vi "GetAcqSeq.vi"(0 "Pre-Looks":i32, 1 "Digitizer Settings":T8={"Digitizer delay (us) "=0.0, "rf points per line"=2048, "lines per plane"=128, "Samp Rate (Hz)"=100000000.0, "Additional dig delay (us)"=0.0, "Voltage Scale"=0.4, "Pre-Looks"=0, "Offset delay (us)"=0.0, "bits A/D"=8, "Avg Num"=1, "DigTimeOut"=5.0, "Rel Dig Delay"=0.0, "Dig Ch"=0, "LeCroyCluster"={"LeCroy Channels"=[TRUE, FALSE, FALSE, FALSE], "LC read pt offset"=0.0, "Sweep Avg"=FALSE}, "Main Digitizer"=enum."NI Digitizer", "Dig Config"=enum."Single channel", "Digitizer ID Cluster"={"Acqiris/Alazar/SP ID"=[], "NI Instr Handles"=[], "LeCroy VISA"="", "GaGe Handle"={"Handle"=0, "Sample size"=0, "Resolution"=0, "Offset"=0, "Channels"=0, "Boards"=0}, "ATS Ref"="ATS9350", "Acqiris Address"=["PCI::INSTR0"], "ADQRef"=refnum, "adq_cu_ptr"=refnum}, "Trigger Settings"={"Trig Source"=1, "Trig Coupling"=0, "Trig Slope"=0, "Level (mV)"=1500.0}, "Bulk Acq"=FALSE, "Bulk Start Indexes"=[], "Data Ref RF"=refnum, "NI ID/Channel"=[], "Total Dig CH"=1, "Xtra Ann Trig delay (us)"=10.0, "Fix Z Delay?"=FALSE, "One Way Transmission?"=FALSE, "Data Ref Log"=refnum} {"Trigger Settings"."Trig Slope" items=["Positive", "Negative"]; "Trigger Settings"."Level (mV)" format="%.2f"; "Trigger Settings"."Trig Coupling" items=["DC 1 MOhm", "AC 1 MOhm", "DC 50 Ohm", "AC 50 Ohm"]; "Trigger Settings"."Trig Source" items=["Chan 1", "External"]; "Rel Dig Delay" format="%.2f"; "DigTimeOut" format="%.2f"; "Avg Num" min=1; "Offset delay (us)" format="%.2f"; "Additional dig delay (us)" format="%.2f"; "Digitizer delay (us)" format="%.2f"}, 3 "Acq Card ID":u32, 6 "Motion Settings":T4={"No Motion?"=FALSE, "Motion System"=enum."NI 735x", "Motion Bd ID"=1, "Motion Profile"="SMAC1", "# Axis"=1, "Reverse Z axis?"=TRUE, "SMAC Axis"=0, "scan pair"=enum."y-(x) scan", "RT fps"=6.0, "Steps per mm"=[1000, 1000, 1000, 1000], "Motor Parameters"={"velocity ct/s"=[10000.0, 10000.0, 10000.0, 50000.0], "accel ct/s^2"=[50000.0, 50000.0, 50000.0, 200000.0]}, "One Way Scan"=FALSE, "Reverse One Way Scan"=FALSE, "Global Position (mm)"=[], "Plane"=0, "Distance between\nscan lines (um)"=0.0, "Distance between\nscan planes (um)"=0.0, "number of scan planes"=1, "Total steps in line"=0, "Xtra plane\ndistance  (um)"=100, "Xtra planes "=1, "Add Axis"=FALSE, "overshoot cts"=200, "BKPT Shift"=0, "Scan Start Time (ms)"=0, "ESP VISA"="GPIB::1::INSTR", "3rd Axis"=1, "GL Ref Out"=refnum, "Galil Address"=""} {"3rd Axis" items=["x", "y", "z", "w"]; "Xtra planes" min=1; "Xtra plane\ndistance  (um)" min=0; "Distance between\nscan planes (um)" format="%.2f"; "Distance between\nscan lines (um)" format="%.2f"; "SMAC Axis" items=["None"=0, "Axis 1"=1, "Axis 2"=2, "Axis 3"=3, "Axis 4"=4, "Axis 5"=5, "Axis 6"=6, "Axis 7"=7, "Axis 8"=8, "Vector Space 1"=17, "Vector Space 2"=18, "Vector Space 3"=19, "Vector Space 4"=20]; "Motion Bd ID" min=1 max=32 step=1}, 7 "errorin":errorcluster, 8 "Numbered File":string, 9 "Divide prf by":i32, 10 "lines per plane":i32, 11 "Channel (1)":i32=1, 12 "Ann Array Params":T1={"Synth Foc?"=FALSE, "Focal Zones"=41, "Switch T/R"=0, "Trans Geometry (mm)"={"Transducer"=0, "Geo Focus"=12.0, "a (radius)"=3.0, "# of rings"=5, "kerf space "=0.1, "Center Freq"=12.0}, "Sub Ap Excite?"=FALSE, "Full Array Scan?"=FALSE, "Xmt/Rcv"={"XMIT"=[TRUE, TRUE, TRUE, TRUE, TRUE], "RCV"=[TRUE, TRUE, TRUE, TRUE, TRUE]}, "PulseSpacing (us)"=0.0, "Xmit Ring"=0, "XMIT CHS"=0, "RCV CHS"=0, "GPU?"=FALSE, "Save TIFF?"=FALSE, "downfactor"=1, "RCV 1CH"=0} {"RCV 1CH" items=["All", "1", "2", "3", "4", "5"]; "Trans Geometry (mm)"."Transducer" items=["6D 12R 40 MHz"=0, "10D 31R 20 MHz"=1, "10D 23R 20 MHz"=2, "6D 23R 40 MHz"=3, "4.5D 10.7R 40 MHz"=4, "9D 23.5R 20 MHz"=5, "9D 25.8R 20MHz"=6, "Enter"=99]; "Switch T/R" min=1 max=5 step=1}, 13 "Rcv Ring":i32, 14 "save?":bool=TRUE, 15 "Reverse?":bool) -> (17 "Raw VGain (scale)":dbl, 18 "Voltage Scale":T12, 20 "Array":i16[][](array[numeric]), 21 "VGain (dB)":dbl, 25 "Synth App Out":i16[][](array[numeric]), 27 "error out":errorcluster)   [LabVIEW 2022 SP3]
uses:
  -DigitizerRoutines/DigitizerSettings.ctl
  -DigitizerRoutines/Digitizer.ctl
  -DigitizerRoutines/DigConfig.ctl
  -DigitizerRoutines/DigitizerID.ctl
  C:/Windows/System32/ADQAPI_dotNet_helper.dll
  Motion Controllers/NI_controller/-NI_MotionRoutines/MotionParameters.ctl
  Motion Controllers/NI_controller/-NI_MotionRoutines/MotionSys.ctl
  Motion Controllers/-MotionRoutines/ScanAxis.ctl
  Motion Controllers/-MotionRoutines/3rdAxis.ctl
  Annular Array/-AnnularRoutines/AnnularArray.ctl
  Annular Array/-AnnularRoutines/TransGeometry.ctl
  Annular Array/-AnnularRoutines/ArrayGeometry.ctl
  VScaleInfoAcq.vi
  Annular Array/-SynthApperture/ProcImageHD_I16.vi
panel:
  # "1-D and 2-D B scan settings"
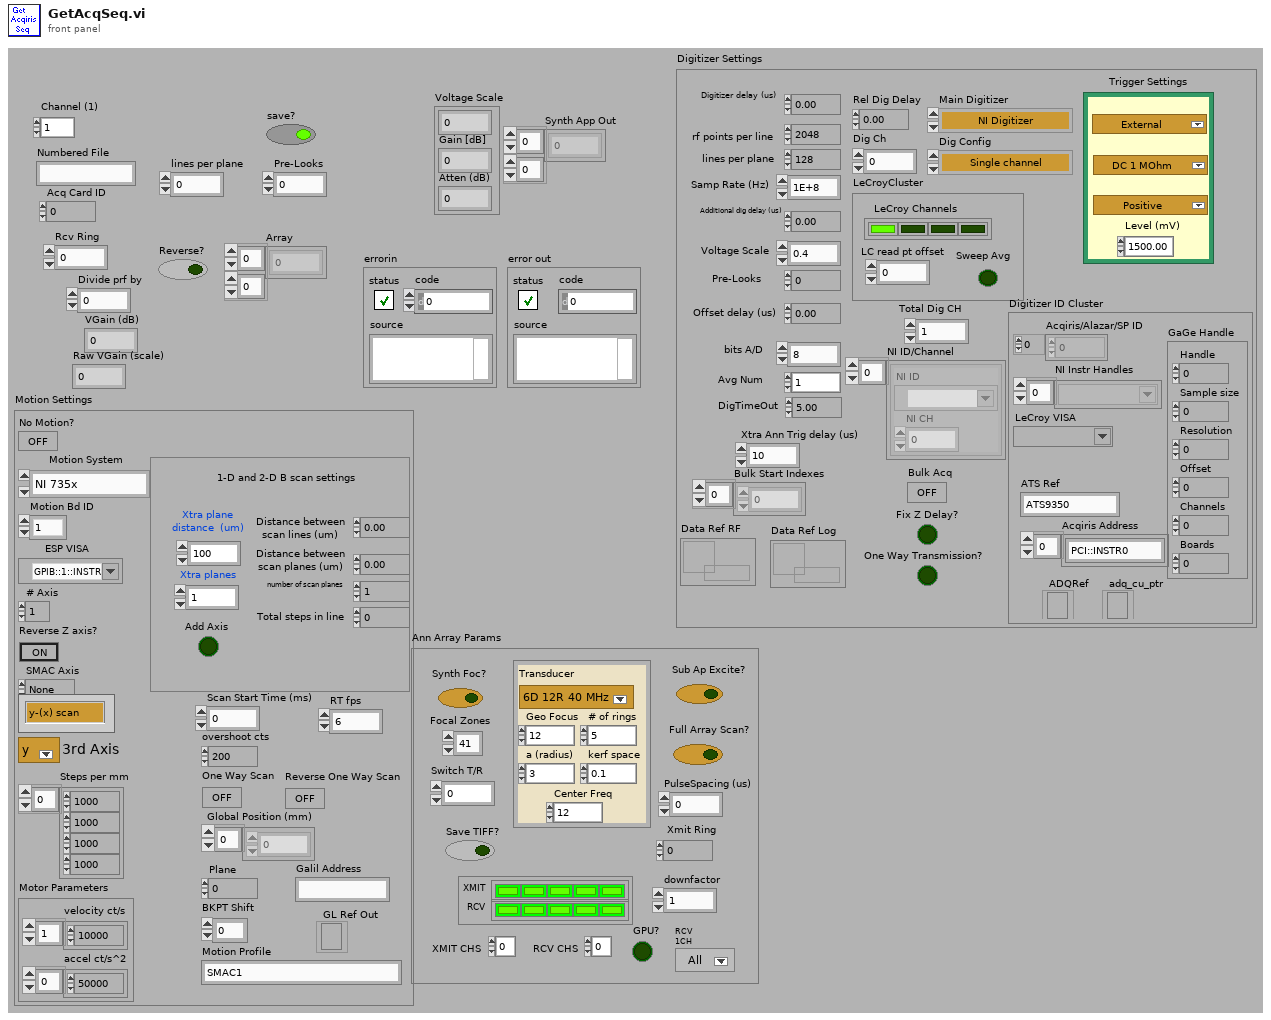
[diagram p1: front panel]
types:
  T1 = typedef "AnnularArray.ctl" = cluster{"Synth Foc?":bool, "Focal Zones":i16, "Switch T/R":i16, "Trans Geometry (mm)":T2, "Sub Ap Excite?":bool, "Full Array Scan?":bool, "Xmt/Rcv":cluster{"XMIT":bool[], "RCV":bool[]}, "PulseSpacing (us)":sgl, "Xmit Ring":i32, "XMIT CHS":u8, "RCV CHS":u8, "GPU?":bool, "Save TIFF?":bool, "downfactor":i32, "RCV 1CH":u16}
  T2 = typedef "TransGeometry.ctl" = cluster{"Transducer":T3, "Geo Focus":dbl, "a (radius)":dbl, "# of rings":i32, "kerf space ":dbl, "Center Freq":dbl}
  T3 = typedef "ArrayGeometry.ctl" = u16
  T4 = typedef "MotionParameters.ctl" = cluster{"No Motion?":bool, "Motion System":T5, "Motion Bd ID":u8, "Motion Profile":string, "# Axis":i8, "Reverse Z axis?":bool, "SMAC Axis":u16, "scan pair":T6, "RT fps":sgl, "Steps per mm":i32[], "Motor Parameters":cluster{"velocity ct/s":dbl[], "accel ct/s^2":dbl[]}, "One Way Scan":bool, "Reverse One Way Scan":bool, "Global Position (mm)":dbl[], "Plane":i32, "Distance between\nscan lines (um)":sgl, "Distance between\nscan planes (um)":sgl, "number of scan planes":i32, "Total steps in line":i32, "Xtra plane\ndistance  (um)":i32, "Xtra planes ":i32, "Add Axis":bool, "overshoot cts":i32, "BKPT Shift":i32, "Scan Start Time (ms)":u32, "ESP VISA":refnum<visa-resource-name>, "3rd Axis":T7, "GL Ref Out":refnum<k7>, "Galil Address":string}
  T5 = typedef "MotionSys.ctl" = enum16{"MM3000", "NI 735x", "Newport ESP", "No Motion Card", "Galil"}
  T6 = typedef "ScanAxis.ctl" = enum16{"y-(x) scan", "x-(y) scan", "z-(x) scan", "z-(y) scan", "y-(z) scan", "x-(z) scan", "w-(x) scan", "w-(y) scan", "w-(z) scan", "x-(w) scan", "y-(w) scan", "z-(w) scan"}
  T7 = typedef "3rdAxis.ctl" = u16
  T8 = typedef "DigitizerSettings.ctl" = cluster{"Digitizer delay (us) ":dbl, "rf points per line":i32, "lines per plane":i32, "Samp Rate (Hz)":dbl, "Additional dig delay (us)":dbl, "Voltage Scale":dbl, "Pre-Looks":i32, "Offset delay (us)":dbl, "bits A/D":i8, "Avg Num":i32, "DigTimeOut":sgl, "Rel Dig Delay":sgl, "Dig Ch":i32, "LeCroyCluster":cluster{"LeCroy Channels":bool[], "LC read pt offset":dbl, "Sweep Avg":bool}, "Main Digitizer":T9, "Dig Config":T10, "Digitizer ID Cluster":T11, "Trigger Settings":cluster{"Trig Source":u16, "Trig Coupling":u16, "Trig Slope":u16, "Level (mV)":dbl}, "Bulk Acq":bool, "Bulk Start Indexes":i32[], "Data Ref RF":refnum<data-value>, "NI ID/Channel":cluster{"NI ID":refnum<k15>, "NI CH":i32}[], "Total Dig CH":i32, "Xtra Ann Trig delay (us)":dbl, "Fix Z Delay?":bool, "One Way Transmission?":bool, "Data Ref Log":refnum<data-value>}
  T9 = typedef "Digitizer.ctl" = enum16{"Acqiris Digitizer", "NI Digitizer", "LeCroy", "GaGe", "AlazarTech", "No Digitizer", "Teledyne"}
  T10 = typedef "DigConfig.ctl" = enum16{"Single channel", "2 Chans w/ 2 Acqiris", "2 Chans w/ 1 Acqiris", "5-CH Pulser New", "5-CH pulser w/ ann array", "5-pass style ann array", "Empty"}
  T11 = typedef "DigitizerID.ctl" = cluster{"Acqiris/Alazar/SP ID":u32[], "NI Instr Handles":refnum<k15>[], "LeCroy VISA":refnum<visa-resource-name>, "GaGe Handle":cluster{"Handle":u32, "Sample size":u32, "Resolution":i32, "Offset":i32, "Channels":u32, "Boards":u32}, "ATS Ref":string, "Acqiris Address":string[], "ADQRef":refnum<k24>, "adq_cu_ptr":refnum<k24>}
  T12 = cluster{sgl, "Gain [dB]  ":sgl, "Atten (dB)":sgl}
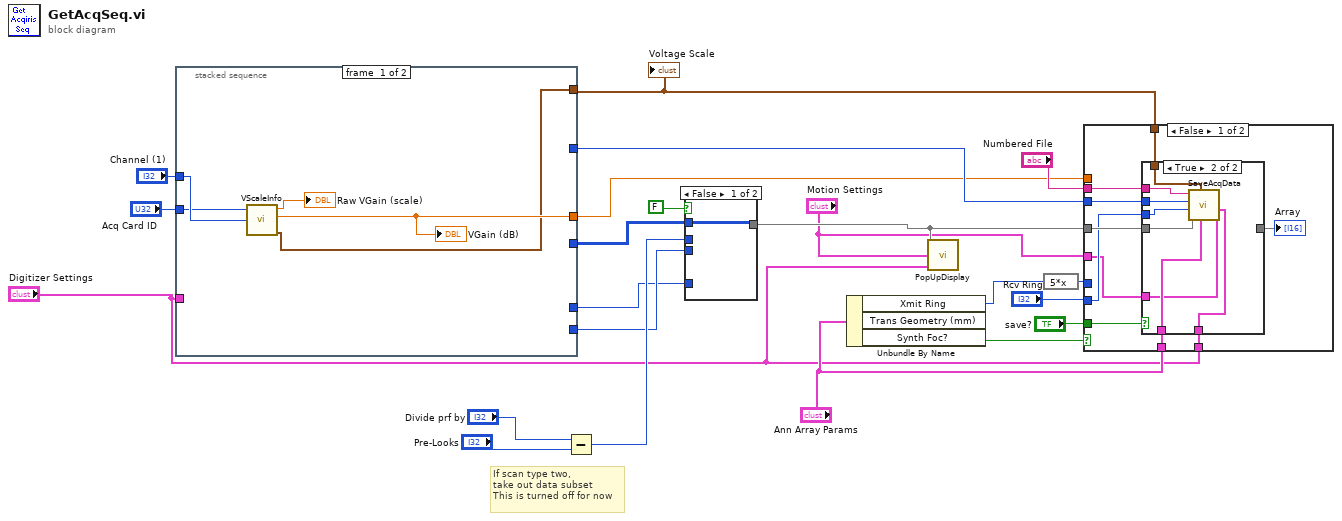
[diagram p0: block diagram]
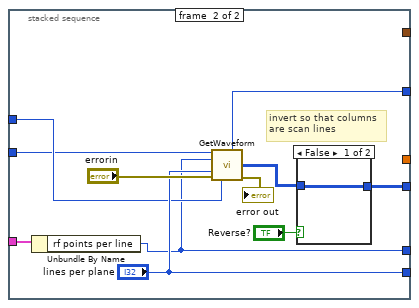
[diagram p2: hidden frame]
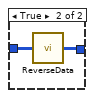
[diagram p3: hidden frame]
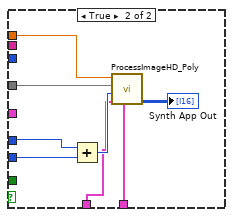
[diagram p5: hidden frame]
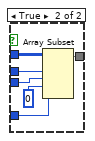
[diagram p6: hidden frame]
diagram:
  # "If scan type two,\ntake out data subset\nThis is turned off for now"
  n1 = stacked-sequence {
    tunnel: [_ w36] -> w19
    tunnel: [_ "lines per plane"] -> w17
    tunnel: [_ w28] -> w16
    tunnel: "Channel (1)" -> [w24 w32]
    tunnel: [_ w30] -> w10
    tunnel: [w26 _] -> w9
    tunnel: "Acq Card ID" -> [w23 w31]
    tunnel: [w25 _] -> w7
    tunnel: "Digitizer Settings" -> [_ w29]
    frame #0 {
      n2 = call-poly "VScaleInfo.vi"("Instrument ID"=w23, "Channel (1)"=w24) -> ("vGain scalar"=→"Raw VGain (scale)":dbl, "vGain (dB)"=w26:dbl, "Voltage Scale"=w25:T12)  [unwired: 1 in, 5 out]
      "VGain (dB)" <- w26
    }
    frame #1 {
      # "invert so that columns\nare scan lines"
      n3 = Unbundle By Name(w29) -> ("rf points per line"=w28:i32)
      n4 = call "GetWaveform.vi"("Acq ID Out"=w31, "Num Samps"=w28, "Num Segs"="lines per plane", "error in"="errorin", "Channel"=w32) -> ("Dig Word Size"=w30:u16, "Acquired Waveform16 bit"=w33:i16[][], "error out"=→"error out":errorcluster)  [unwired: 1 in, 7 out]
      n5 = case shown="False" "Reverse?" {
        tunnel: w33 -> [w39 w41]
        tunnel: [w39 w40] -> w36
        frame False {
        }
        frame True {
          n6 = call "ReverseData.vi"("Array in"=w41) -> ("Array out"=w40:i16[][])
        }
      }
    }
  }
  "Voltage Scale" <- w7
  n7 = Subtract(x="Divide prf by", y="Pre-Looks") -> (x-y=w21:i32)
  n8 = case shown="False" FALSE {
    tunnel: w19 -> [w42 w48]
    tunnel: [w42 w47] -> w3
    tunnel: w17 -> [_ w46]
    tunnel: w16 -> [_ w45]
    tunnel: w21 -> [_ w43]
    frame False {
    }
    frame True {
      n9 = Array Subset(array=w48, index (row)=w43, length (row)=w46, index (col)=0, length (col)=w45) -> (w47:i16[][])
    }
  }
  n10 = Unbundle By Name("Ann Array Params") -> ("Xmit Ring"=w4:i32, "Synth Foc?"=w6:bool)  [unwired: 1 out]
  n11 = call "PopUpDisplay.vi"("Data"=w3, "Motion Settings In"="Motion Settings", "Digitizer Settings"="Digitizer Settings") -> ()  [unwired: 13 in]
  n12 = expression code="5*x"(w4) -> (w15:i32)
  n13 = case shown="False" w6 {
    tunnel: w10 -> [w58 _]
    tunnel: "save?" -> [w57 _]
    tunnel: w3 -> [w56 w75]
    tunnel: w15 -> [_ w74]
    tunnel: "Numbered File" -> [w55 _]
    tunnel: "Rcv Ring" -> [w51 w72]
    tunnel: w9 -> [_ w71]
    tunnel: w7 -> [w53 _]
    tunnel: "Digitizer Settings" -> [w52 w69]
    tunnel: "Ann Array Params" -> [w50 w68]
    tunnel: "Motion Settings" -> [w49 _]
    frame False {
      n14 = case shown="True" w57 {
        tunnel: w58 -> [_ w67]
        tunnel: w56 -> [w59 w66]
        tunnel: [w59 _] -> w54
        tunnel: w55 -> [_ w65]
        tunnel: w53 -> [_ w64]
        tunnel: w52 -> [_ w63]
        tunnel: w51 -> [_ w62]
        tunnel: w50 -> [_ w61]
        tunnel: w49 -> [_ w60]
        frame False {
        }
        frame True {
          n15 = call "SaveAcqData.vi"("Digitizer Settings"=w63, "Motion Settings"=w60, "Ann Array Params"=w61, "Votage scaling"=w64, "Array"=w66, "Pulser Channel"=w62, "Dig Word Size"=w67, "File Name"=w65) -> ()  [unwired: 3 in]
        }
      }
      "Array" <- w54
    }
    frame True {
      n16 = Add(x=w74, y=w72) -> (x+y=w73:i32)
      n17 = call-poly "ProcessImageHD_Poly.vi"("Digitizer Settings"=w69, "Ann Array Params"=w68, "T/R Ring"=w73, "Scan Data In"=w75, "Att (dB)"=w71) -> ("Synth App Out"=→"Synth App Out":i16[][])  [unwired: 3 in, 1 out]
    }
  }
